vi "Update Point Data.vi"(9 "Data":variant, 10 "Point Ident":string, 11 "Task Actor in":refnum<class "Task Actor.lvclass">) -> (3 "Task Actor out":refnum<class "Task Actor.lvclass">)   [LabVIEW 2024, in "Task Actor.lvlib" / "Task Actor.lvclass"]
uses:
  Task Actor.lvclass
  Task Actor.lvclass/Task Actor.ctl
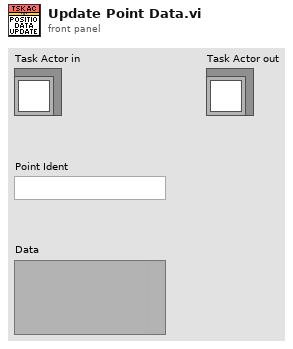
[diagram p1: front panel]
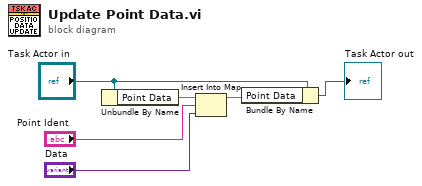
[diagram p0: block diagram]
diagram:
  n1 = Unbundle By Name("Task Actor in") -> ("Point Data"=w4:map{string, variant})
  n2 = Insert Into Map(map in=w4, key="Point Ident", value="Data") -> (map out=w3:map{string, variant})  [unwired: 2 out]
  n3 = Bundle By Name(cluster="Task Actor in", "Point Data"=w3) -> (→"Task Actor out":refnum<class "Task Actor.lvclass">)
